vi "Read Setpoint (Single).vi"(8 "error in":errorcluster, 9 "Channel Index":i32=1, 11 "Setpoint.lvclass":refnum<class "Setpoint.lvclass">) -> (0 "error out":errorcluster, 1 "Changed or First Call?":bool, 2 "Current Setpoint":dbl, 3 "Setpoint.lvclass 2":refnum<class "Setpoint.lvclass">)   [LabVIEW 2023, in "Setpoint.lvclass"]
uses:
  Setpoint.lvclass
  Setpoint.lvclass/Setpoint.ctl
  <vilib>/ADAS Replay HIL/Channels/Tag Wrapper/Polymorphic/Read Channel (Double).vi
  b4f2a3c3-1a4a-4d01-ae5f-fb73a1936019.vi
  <vilib>/ADAS Replay HIL/Channels/Tag Wrapper/Polymorphic/Read Channel (Double).vi/b2f764de-0c1e-4784-a155-687fc995a684.vi
  <vilib>/ADAS Replay HIL/Channels/Tag Wrapper/Polymorphic/Read Channel (Double).vi/b2f764de-0c1e-4784-a155-687fc995a684.vi/c28b0ead-42ad-4072-80a2-aca7f2bd7ce3.vi
  <vilib>/ADAS Replay HIL/Channels/Tag Wrapper/Polymorphic/Read Channel (Double).vi/b2f764de-0c1e-4784-a155-687fc995a684.vi/219d0231-d98b-4193-b5cc-84f90e3c9091.vi
  <vilib>/ADAS Replay HIL/Channels/Tag Wrapper/Tag Wrapper.lvlib
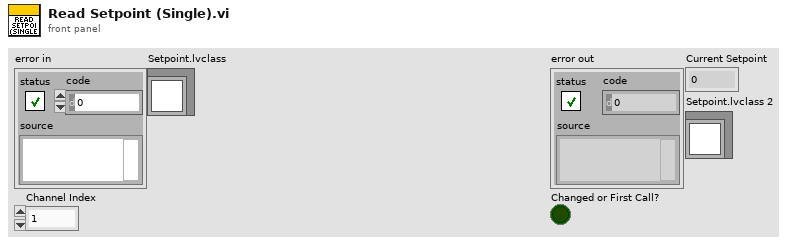
[diagram p1: front panel]
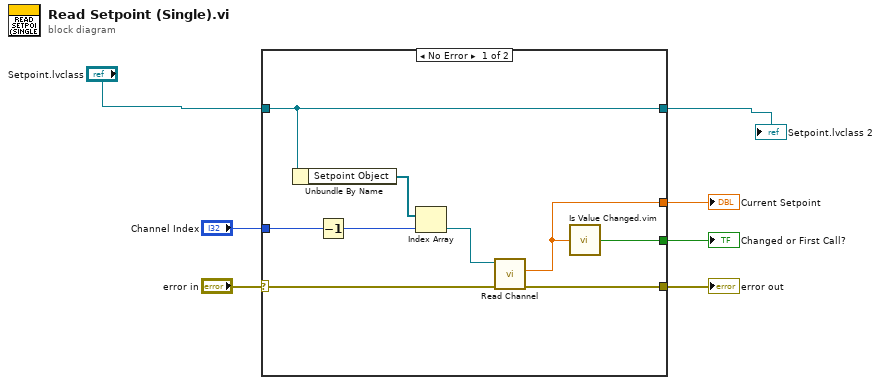
[diagram p0: block diagram]
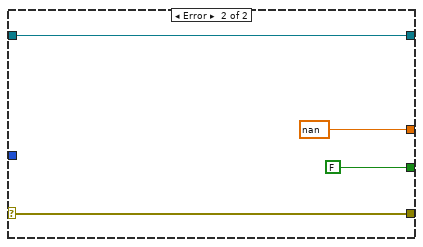
[diagram p2: hidden frame]
diagram:
  n1 = case shown="No Error" "error in" {
    selector: "error in" -> [w14 w20]
    tunnel: [w13 w20] -> w6
    tunnel: [w16 w19] -> w5
    tunnel: "Setpoint.lvclass" -> [w16 w19]
    tunnel: [w12 nan] -> w3
    tunnel: [w11 FALSE ("changed or first call?")] -> w4
    tunnel: "Channel Index" -> [w9 _]
    frame No Error {
      n2 = Unbundle By Name(w16) -> ("Setpoint Object"=w15:refnum<k21>[])
      n3 = Decrement(x=w9) -> (x-1=w8:i32)
      n4 = Index Array(array=w15, index=w8) -> (element=w10:refnum<k21>)
      n5 = call-poly <vilib>:"Read Channel.vi"("error in"=w14, "ADAS HIL Channel in"=w10) -> ("error out"=w13:errorcluster, "Value out"=w12:dbl)  [unwired: 6 in, 2 out]
      n6 = call "Is Value Changed.vim"("value"=w12) -> ("changed or first call?"=w11:bool)
    }
    frame Error {
    }
  }
  "error out" <- w6
  "Changed or First Call?" <- w4
  "Current Setpoint" <- w3
  "Setpoint.lvclass 2" <- w5
